vi "Y scale properties.vi"(8 "Min":string[](array[string]), 9 "Max":string[](array[string]), 10 "Active index":i32, 11 "XYGraph in":refnum<vi>) -> ()   [LabVIEW 2020]
doc: "This vi scales the graph y scale as per min and max values\nIf min and max values not available then autoscale is ON\ninput\n1.Active index for graph plot\n2. max values array\n3. min values array"
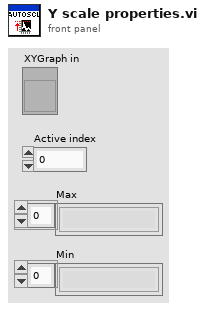
[diagram p1: front panel]
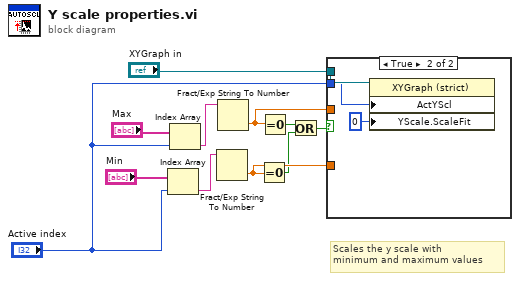
[diagram p0: block diagram]
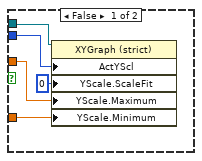
[diagram p2: hidden frame]
diagram:
  # "Scales the y scale with \nminimum and maximum values"
  n1 = Index Array(array="Min", index="Active index") -> (element=w9:string)
  n2 = Index Array(array="Max", index="Active index") -> (element=w8:string)
  n3 = Fract/Exp String To Number(string=w9) -> (number=w5:dbl)  [unwired: 3 in, 1 out]
  n4 = Fract/Exp String To Number(string=w8) -> (number=w4:dbl)  [unwired: 3 in, 1 out]
  n5 = Equal To 0?(x=w5) -> (x = 0?=w2:bool)
  n6 = Equal To 0?(x=w4) -> (x = 0?=w1:bool)
  n7 = Or(x=w1, y=w2) -> (x .or. y?=w3:bool)
  n8 = case shown="True" w3 {
    tunnel: w4 -> [w16 _]
    tunnel: w5 -> [w15 _]
    tunnel: "Active index" -> [w12 w17]
    tunnel: "XYGraph in" -> [w13 w19]
    frame False {
      n9 = property class="XYGraph (strict)"(reference=w13, "ActYScl"=w12, "YScale.ScaleFit"=u8 0 ("Y Scale.Scale Fit"), "YScale.Maximum"=w16, "YScale.Minimum"=w15) -> ()  [unwired: 1 in, 2 out]
    }
    frame True {
      n10 = property class="XYGraph (strict)"(reference=w19, "ActYScl"=w17, "YScale.ScaleFit"=u8 0 ("Y Scale.Scale Fit")) -> ()  [unwired: 1 in, 2 out]
    }
  }
